vi "ServiceChannels.GetRefs.vi"(8 "error in (no error)":errorcluster, 11 "Item Ref in":T1 format="%.0x") -> (0 "error out":errorcluster, 1 "Status":T1[](array[typedef]) format="%.0x", 2 "Trigger":T1[](array[typedef]) format="%.0x", 3 "Section Ref out":T1 format="%.0x")   [LabVIEW 2019, in "Diagnostics Addon System Explorer.lvlib"]
uses:
  <vilib>/NI VeriStand/Custom Device API/Custom Device Item Ref.ctl
  Shared/SubVIs/Constants.vi
  <vilib>/NI VeriStand/Custom Device Tools/Custom Device Utility Library/NI VeriStand - Search for Item by GUID.vi
  <vilib>/NI VeriStand/Custom Device Tools/Custom Device Utility Library/NI VeriStand - Search for Item by Name.vi
  Diagnostics Addon System Explorer.lvlib
  <vilib>/NI VeriStand/Custom Device Tools/Custom Device Utility Library/Custom Device Utility Library.lvlib
  Shared/Diagnostics Addon Shared.lvlib
  <vilib>/NI VeriStand/Custom Device API/Custom Device API.lvlib
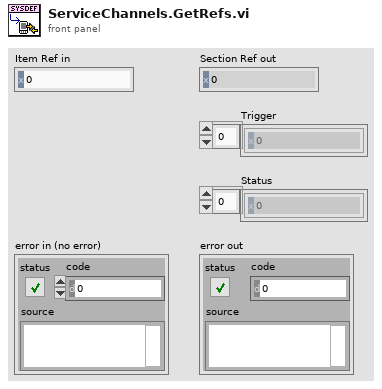
[diagram p1: front panel]
types:
  T1 = typedef "Custom Device API.lvlib/Custom Device Item Ref.ctl" = u64
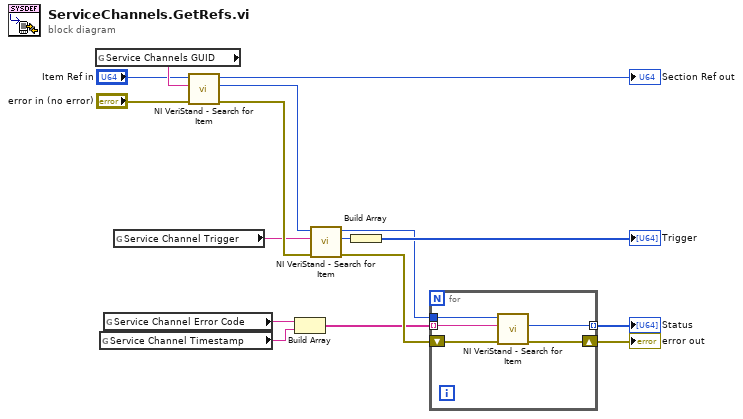
[diagram p0: block diagram]
diagram:
  n1 = global read "Constants.vi" "Service Channels GUID"() -> (w4:string)
  n2 = global read "Constants.vi" "Service Channel Timestamp"() -> (w8:string)
  n3 = global read "Constants.vi" "Service Channel Error Code"() -> (w7:string)
  n4 = global read "Constants.vi" "Service Channel Trigger"() -> (w6:string)
  n5 = call-poly <vilib>:"NI VeriStand - Search for Item.vi"("error in"="error in (no error)", "Item GUID"=w4, "Section Ref in"="Item Ref in") -> ("error out"=w14:errorcluster, "Item Ref"=w5:T1, "Section Ref out"=→"Section Ref out":T1)  [unwired: 5 in, 1 out]
  n6 = Build Array(w7, w8) -> (w9:string[])
  n7 = call-poly <vilib>:"NI VeriStand - Search for Item.vi"("error in"=w14, "Item Name"=w6, "Section Ref in"=w5) -> ("error out"=w10:errorcluster, "Item Ref"=w12:T1, "Section Ref out"=w11:T1)  [unwired: 5 in, 1 out]
  n8 = Build Array(w12) -> (→"Trigger":T1[])
  n9 = for {
    tunnel: w9 -> [w21] mode=indexing
    shift-right: [w19] -> w15
    shift-left: w10 -> [w20]
    tunnel: w11 -> [w18]
    tunnel: [w17] -> w13 mode=indexing
    n10 = call-poly <vilib>:"NI VeriStand - Search for Item.vi"("error in"=w20, "Item Name"=w21, "Section Ref in"=w18) -> ("error out"=w19:errorcluster, "Item Ref"=w17:T1)  [unwired: 5 in, 2 out]
  }
  "error out" <- w15
  "Status" <- w13
